vi "Start or Get Execution.vi"() -> (6 "Execution Events":T1)   [LabVIEW 2022 SP3, in "FlexBlocks Support.lvlib"]
uses:
  FlexBlocks Support.lvlib
  Block State.ctl
  Block Phase.ctl
  Block Status.ctl
  Block Status with Error.ctl
  Block Command.ctl
  Worker Block.ctl
  Worker Registration.ctl
  Execution Events.ctl
  <extravilib>/ChannelInstances/Flex-t'FlexBlocks Support.lvlib-Execution Events.ctl'.lvlib
  <extravilib>/ChannelInstances/Flex-t'FlexBlocks Support.lvlib-Execution Events.ctl'/))Channel.ctl
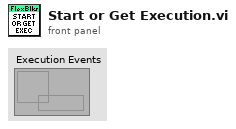
[diagram p1: front panel]
types:
  T1 = typedef "Flex-t'FlexBlocks Support.lvlib-Execution Events.ctl'.lvlib/))Channel.ctl" = refnum<queue>
  T2 = typedef "FlexBlocks Support.lvlib/Execution Events.ctl" = cluster{"Registration":refnum<user-event>, "Init":refnum<user-event>, "Run":refnum<user-event>, "Step":refnum<user-event>, "Stop":refnum<user-event>, "Close":refnum<user-event>, "Block Status":refnum<user-event>}
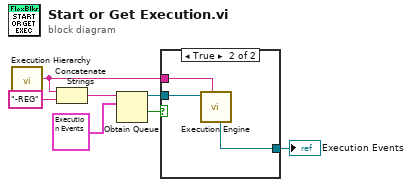
[diagram p0: block diagram]
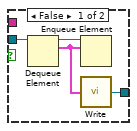
[diagram p2: hidden frame]
diagram:
  n1 = call "Execution Hierarchy.vi"() -> ("Top Level VI Name"=w3:string)  [unwired: 11 in]
  n2 = Concatenate Strings(w3, "-REG" ("string")) -> (w6:string)
  n3 = Obtain Queue(name (unnamed)=w6, element data type=T2 {"Registration"=refnum, "Init"=refnum, "Run"=refnum, "Step"=refnum, "Stop"=refnum, "Close"=refnum, "Block Status"=refnum} ("Execution Events")) -> (queue out=w4:refnum<queue>, created new?=w5:bool)  [unwired: 3 in, 1 out]
  n4 = case shown="True" w5 {
    tunnel: w4 -> [w11 w12]
    tunnel: w3 -> [_ w14]
    tunnel: [w8 w13] -> w1
    frame False {
      n5 = Dequeue Element(queue=w11) -> (queue out=w10:refnum<queue>, element=w9:T2)  [unwired: 2 in, 2 out]
      n6 = Enqueue Element(queue=w10, element=w9) -> ()  [unwired: 2 in, 3 out]
      n7 = call <extravilib>:"Write.vi"("element"=w9) -> ("channel"=w8:T1)  [unwired: 6 in, 2 out]
    }
    frame True {
      n8 = call "Execution Engine.vi"("Execution Events"=w13, "Hierarchy"=w14, "Reg Event Queue"=w12) -> ()  [unwired: 9 in]
    }
  }
  "Execution Events" <- w1
